vi "reprGraphical.vi"(8 "error in (no error)":errorcluster, 9 "Image Descriptor":T1={"Upper-Left Corner Coordinates"={"UTM Zone"=0.0, "Hemisphere"=enum."North", "East"=0.0, "North"=0.0}, "Meters/Pixel"=42.294203} {"Upper-Left Corner Coordinates"."North" format="%#_10f"; "Upper-Left Corner Coordinates"."East" format="%#_8f"}, 10 "Image In":T3, 11 "PassBuoys in":refnum<class "PassBuoys.lvclass">) -> (0 "error out":errorcluster, 2 "Image Out":T3, 3 "PassBuoys out":refnum<class "PassBuoys.lvclass">)   [LabVIEW 2011, in "PassBuoys.lvclass"]
doc: "Draws the two buoys on the mission map. The Image Descriptor and the PassBuoys have relative positions to each other. Once this is determined, the waypoint symbols are drawn on the map at their locations on the map image, relative to the GPS coordinates of the map."
uses:
  PassBuoys.lvclass
  <vilib>/vision/Image Controls.llb/IMAQ Image.ctl
  0-OCU/0 Code/mission input/0-Image Descriptor.ctl
  2 Typedefs/UTM Location.ctl
  PassBuoys.lvclass/PassBuoys.ctl
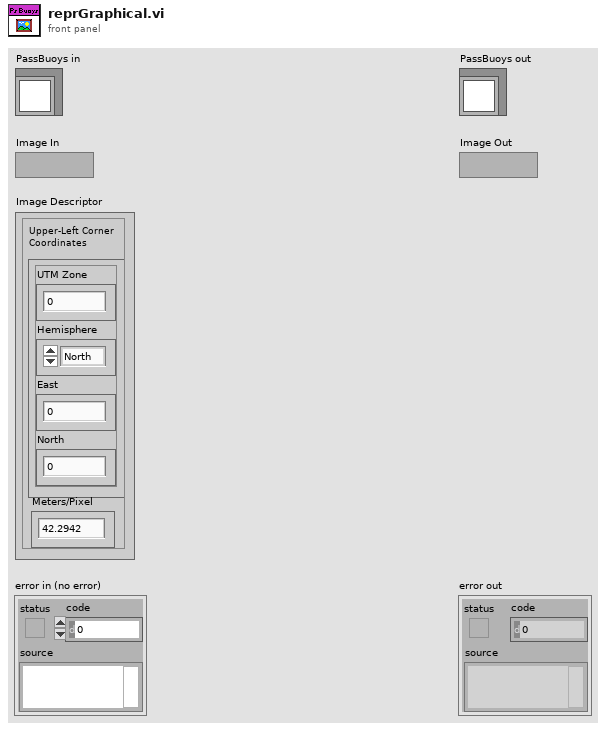
[diagram p1: front panel]
types:
  T1 = typedef "0-Image Descriptor.ctl" = cluster{"Upper-Left Corner Coordinates":T2, "Meters/Pixel":dbl}
  T2 = typedef "UTM Location.ctl" = cluster{"UTM Zone":dbl, "Hemisphere":enum16{"North", "South"}, "East":dbl, "North":dbl}
  T3 = typedef "IMAQ Image.ctl" = refnum<image>
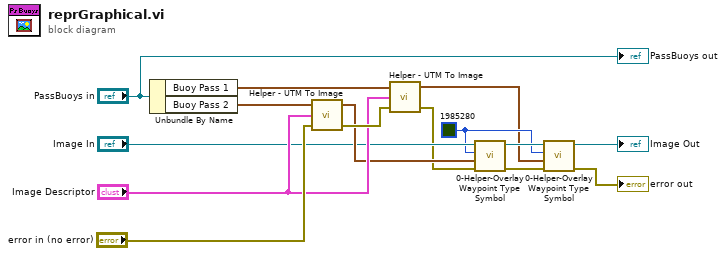
[diagram p0: block diagram]
diagram:
  w2 = u32 1985280 ("Icon Color")
  n1 = Unbundle By Name("PassBuoys in") -> ("Buoy Pass 1"=w14:T2, "Buoy Pass 2"=w15:T2)
  n2 = call "Helper - UTM To Image.vi"("error in"="error in (no error)", "Image Descriptor"="Image Descriptor", "UTM Location"=w15) -> ("error out"=w12:errorcluster, "Pixel Coordinates"=w10:cluster{"X":i32, "Y":i32})  [unwired: 1 out]
  n3 = call "Helper - UTM To Image.vi"("error in"=w12, "Image Descriptor"="Image Descriptor", "UTM Location"=w14) -> ("error out"=w8:errorcluster, "Pixel Coordinates"=w1:cluster{"X":i32, "Y":i32})  [unwired: 1 out]
  n4 = call "0-Helper-Overlay Waypoint Type Symbol.vi"("error in"=w8, "Overlay Location"=w10, "Icon Color"=w2, "Image in"="Image In") -> ("error out"=w5:errorcluster, "Image out"=w6:T3)  [unwired: 6 in]
  n5 = call "0-Helper-Overlay Waypoint Type Symbol.vi"("error in"=w5, "Overlay Location"=w1, "Icon Color"=w2, "Image in"=w6) -> ("error out"=→"error out":errorcluster, "Image out"=→"Image Out":T3)  [unwired: 6 in]
  "PassBuoys out" <- "PassBuoys in"
